vi "Flatten to YAML.vi"(4 "Condensed?":bool, 6 "No Label?":bool, 8 "error in (no error)":errorcluster, 11 "YAML Parser in":refnum<class "YAML Parser.lvclass">) -> (0 "error out":errorcluster, 2 "YAML String":string, 3 "YAML Parser out":refnum<class "YAML Parser.lvclass">)   [LabVIEW 2015, in "YAML Parser.lvclass"]
uses:
  YAML Parser.lvclass
  YAML Parser.lvclass/YAML Parser.ctl
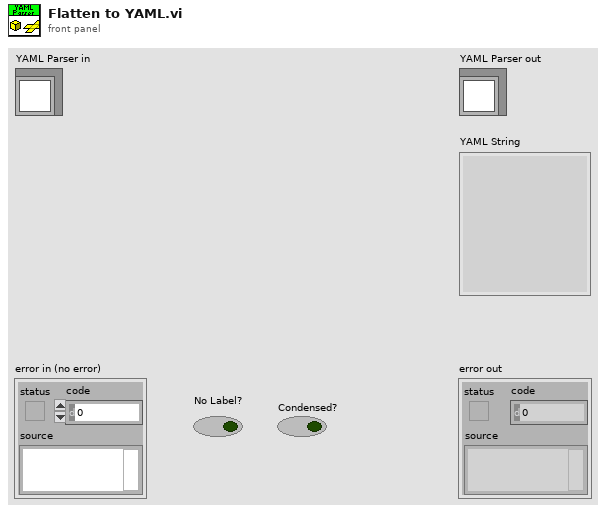
[diagram p1: front panel]
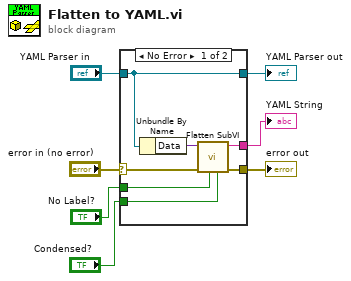
[diagram p0: block diagram]
diagram:
  n1 = case shown="No Error" "error in (no error)" {
    selector: "error in (no error)" -> [w14 w16]
    tunnel: [w13 w16] -> w6
    tunnel: [w12 w15] -> w4
    tunnel: "YAML Parser in" -> [w12 w15]
    tunnel: [w10 _] -> w3
    tunnel: "No Label?" -> [w9 _]
    tunnel: "Condensed?" -> [w8 _]
    frame No Error {
      n2 = Unbundle By Name(w12) -> ("Data"=w11:variant)
      n3 = call "Flatten SubVI.vi"("Condensed?"=w8, "No Label?"=w9, "error in (no error)"=w14, "Data"=w11) -> ("error out"=w13:errorcluster, "YAML String out"=w10:string)  [unwired: 6 in]
    }
    frame Error {
    }
  }
  "error out" <- w6
  "YAML Parser out" <- w4
  "YAML String" <- w3
